vi "tailflickgui_v0.3.vi"() -> ()   [LabVIEW 2011]
uses:
  <vilib>/Utility/error.llb/DialogType.ctl
  <vilib>/Instr/_visa.llb/VISA Flush IO Buffer Mask.ctl
  <vilib>/Instr/_visa.llb/VISA Configure Serial Port (Instr).vi
  <vilib>/Utility/file.llb/Write To Spreadsheet File (string).vi
panel:
  in  "Start?":bool
  in  "End Experiments?":bool
  out "find list":string[](array[string])
  out "VISA resource name out":refnum<visa-resource-name>
  out "Lamp On":bool
  out "Elapsed Time (s)":dbl
  out "new file path (Not A Path if cancelled)":path
  in  "Sample Name":string="Mouse1"
  in  "Filename":path
  out "Start ms":u32
  out "Data Bits":u32
  in  "Arduino Port":refnum<visa-resource-name>
  in  "Baud Rate":dbl=19200.0
  out "USB Output":string
  out "error out":errorcluster
  in  "error in (no error)":errorcluster
  # "Important inputs and outputs for the user."
  # "Inputs and Outputs that should not need to be changed. They are for debugging."
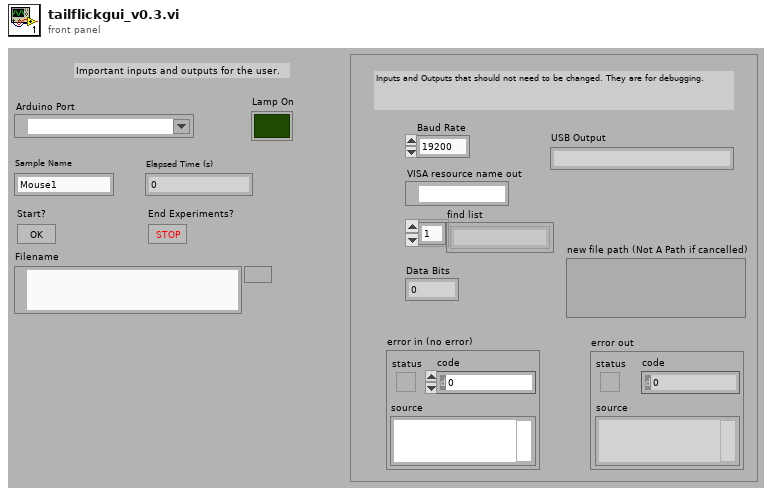
[diagram p1: front panel]
types:
  T1 = typedef "DialogType.ctl" = u16
  T2 = typedef "VISA Flush IO Buffer Mask.ctl" = u16
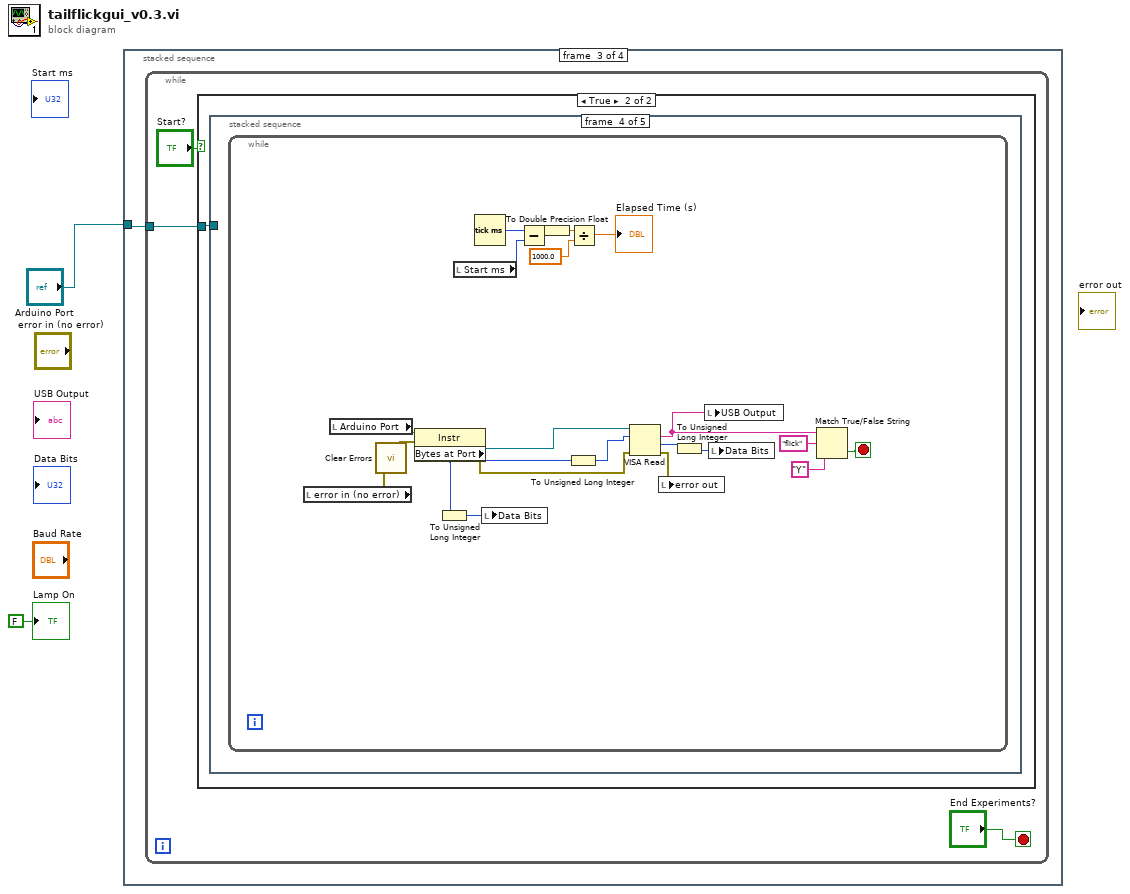
[diagram p0: block diagram]
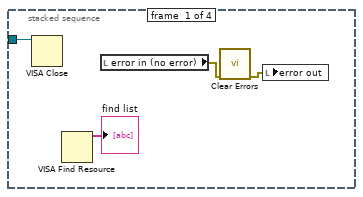
[diagram p2: hidden frame]
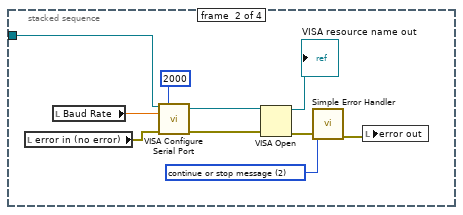
[diagram p3: hidden frame]
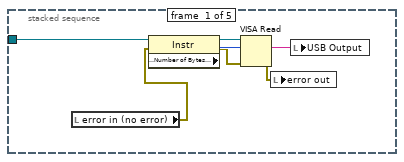
[diagram p5: hidden frame]
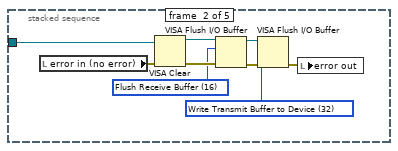
[diagram p6: hidden frame]
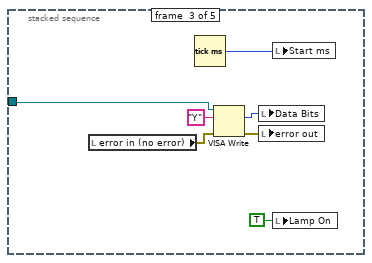
[diagram p7: hidden frame]
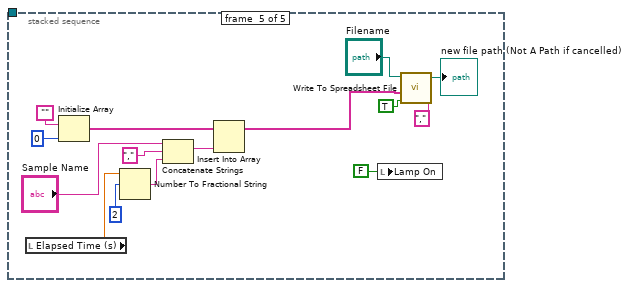
[diagram p8: hidden frame]
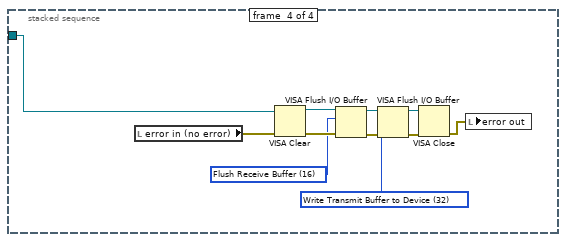
[diagram p9: hidden frame]
diagram:
  n1 = stacked-sequence {
    tunnel: "Arduino Port" -> [w4 w13 w17 w81]
    frame #0 {
      n2 = VISA Close(VISA resource name=w4) -> ()  [unwired: 1 in, 1 out]
      n3 = VISA Find Resource() -> (3:→"find list":string[])  [unwired: 3 in, 2 out]
      n4 = local read "error in (no error)"() -> (w6:errorcluster)
      n5 = call <vilib>:"Clear Errors.vi"("error in (no error)"=w6) -> ("error out"=w5:errorcluster)  [unwired: 6 in]
      n6 = local write "error out"(w5) -> ()
    }
    frame #1 {
      w8 = T1 2 items=["no dialog", "OK message", "continue or stop message", "OK message + warnings", "continue/stop + warnings"] ("type of dialog (OK msg:1)")
      n7 = local read "error in (no error)"() -> (w14:errorcluster)
      n8 = local read "Baud Rate"() -> (w16:dbl)
      n9 = call-poly "VISA Configure Serial Port"("VISA resource name"=w13, "timeout (10sec)"=u32 2000, "baud rate (9600)"=w16, "error in (no error)"=w14) -> ("VISA resource name out"=w12:refnum<visa-resource-name>, "error out"=w11:errorcluster)  [unwired: 10 in]
      n10 = VISA Open(error in (no error)=w11, VISA resource name=w12) -> (VISA resource name=→"VISA resource name out":refnum<visa-resource-name>, error out=w10:errorcluster)  [unwired: 3 in]
      n11 = call <vilib>:"Simple Error Handler.vi"("type of dialog (OK msg:1)"=w8, "error in (no error)"=w10) -> ("error out"=w9:errorcluster)  [unwired: 3 in, 4 out]
      n12 = local write "error out"(w9) -> ()
    }
    frame #2 {
      n13 = while {
        tunnel: w17 -> [w18]
        stop <- "End Experiments?" stop-if-true
        n14 = case shown="True" "Start?" {
          tunnel: w18 -> [_ w21]
          frame False {
          }
          frame True {
            n15 = stacked-sequence {
              tunnel: w21 -> [w25 w29 w40 _ _]
              frame #0 {
                n16 = local read "error in (no error)"() -> (w22:errorcluster)
                n17 = property class="Instr"(reference=w25, error in=w22) -> (reference out=w24:refnum<visa-resource-name>, error out=w23:errorcluster, "Serial Settings:Number of Bytes at Serial Port"=w26:u32)
                n18 = VISA Read(VISA resource name=w24, byte count=w26, error in (no error)=w23) -> (read buffer=w27:string, error out=w28:errorcluster)  [unwired: 2 out]
                n19 = local write "error out"(w28) -> ()
                n20 = local write "USB Output"(w27) -> ()
              }
              frame #1 {
                w33 = T2 32 items=["Flush Receive Buffer"=16, "Write Transmit Buffer to Device"=32, "Flush Receive Buffer (No I/O)"=64, "Flush Transmit Buffer"=128] ("Mask")
                w35 = T2 16 items=["Flush Receive Buffer"=16, "Write Transmit Buffer to Device"=32, "Flush Receive Buffer (No I/O)"=64, "Flush Transmit Buffer"=128] ("Mask")
                n21 = local read "error in (no error)"() -> (w30:errorcluster)
                n22 = VISA Clear(VISA resource name=w29, error in (no error)=w30) -> (VISA resource name out=w36:refnum<visa-resource-name>, error out=w37:errorcluster)
                n23 = VISA Flush I/O Buffer(VISA resource name=w36, mask (16)=w35, error in (no error)=w37) -> (VISA resource name out=w32:refnum<visa-resource-name>, error out=w34:errorcluster)
                n24 = VISA Flush I/O Buffer(VISA resource name=w32, mask (16)=w33, error in (no error)=w34) -> (error out=w31:errorcluster)  [unwired: 1 out]
                n25 = local write "error out"(w31) -> ()
              }
              frame #2 {
                n26 = local read "error in (no error)"() -> (w43:errorcluster)
                n27 = Tick Count (ms)() -> (millisecond timer value=w38:u32)
                n28 = VISA Write(VISA resource name=w40, write buffer="Y", error in (no error)=w43) -> (return count=w41:u32, error out=w42:errorcluster)  [unwired: 1 out]
                n29 = local write "Data Bits"(w41) -> ()
                n30 = local write "error out"(w42) -> ()
                n31 = local write "Start ms"(w38) -> ()
                n32 = local write "Lamp On"(TRUE) -> ()
              }
              frame #3 {
                n33 = while {
                  stop <- w60 stop-if-true
                  n34 = local read "error in (no error)"() -> (w56:errorcluster)
                  n35 = local read "Arduino Port"() -> (w55:refnum<visa-resource-name>)
                  n36 = call <vilib>:"Clear Errors.vi"("error in (no error)"=w56) -> ("error out"=w54:errorcluster)  [unwired: 6 in]
                  n37 = property class="Instr"(reference=w55, error in=w54) -> (reference out=w63:refnum<visa-resource-name>, error out=w61:errorcluster, "Bytes at Port"=w62:u32)
                  n38 = To Unsigned Long Integer(number=w62) -> (unsigned 32bit integer=w51:u32)
                  n39 = local read "Start ms"() -> (w48:u32)
                  n40 = Tick Count (ms)() -> (millisecond timer value=w50:u32)
                  n41 = local write "Data Bits"(w51) -> ()
                  n42 = Subtract(x=w50, y=w48) -> (x-y=w49:u32)
                  n43 = To Double Precision Float(number=w49) -> (double precision float=w45:dbl)
                  n44 = To Unsigned Long Integer(number=w62) -> (unsigned 32bit integer=w53:u32)
                  n45 = Divide(x=w45, y=1000.0) -> (x/y=→"Elapsed Time (s)":dbl)
                  n46 = VISA Read(VISA resource name=w63, byte count=w53, error in (no error)=w61) -> (read buffer=w64:string, return count=w59:u32, error out=w57:errorcluster)  [unwired: 1 out]
                  n47 = local write "error out"(w57) -> ()
                  n48 = To Unsigned Long Integer(number=w59) -> (unsigned 32bit integer=w52:u32)
                  n49 = local write "USB Output"(w64) -> ()
                  n50 = local write "Data Bits"(w52) -> ()
                  n51 = Match True/False String(2:"Y" ("false string"), 3:"flick" ("true string"), 4:w64) -> (0:w60:bool)  [unwired: 1 out]
                }
              }
              frame #4 {
                n52 = local read "Elapsed Time (s)"() -> (w68:dbl)
                n53 = Initialize Array("", 0 ("index")) -> (w74:string[])
                n54 = Number To Fractional String(number=w68, width (-)=i16 2 ("precision (6)")) -> (F-format string=w70:string)  [unwired: 2 in]
                n55 = Concatenate Strings("Sample Name", ",", w70) -> (w72:string)
                n56 = Insert Into Array(array=w74, new element=w72) -> (w67:string[])  [unwired: 1 in]
                n57 = local write "Lamp On"(FALSE ("Lamp On")) -> ()
                n58 = call-poly <vilib>:"Write To Spreadsheet File.vi"("delimiter (\\t)"="," ("delimiter (\\t)"), "append to file? (new file:F)"=TRUE, "1D data"=w67, "file path (dialog if empty)"="Filename") -> ("new file path (Not A Path if cancelled)"=→"new file path (Not A Path if cancelled)":path)  [unwired: 4 in]
              }
            }
          }
        }
      }
    }
    frame #3 {
      w87 = T2 32 items=["Flush Receive Buffer"=16, "Write Transmit Buffer to Device"=32, "Flush Receive Buffer (No I/O)"=64, "Flush Transmit Buffer"=128] ("Mask")
      w89 = T2 16 items=["Flush Receive Buffer"=16, "Write Transmit Buffer to Device"=32, "Flush Receive Buffer (No I/O)"=64, "Flush Transmit Buffer"=128] ("Mask")
      n59 = local read "error in (no error)"() -> (w85:errorcluster)
      n60 = VISA Clear(VISA resource name=w81, error in (no error)=w85) -> (VISA resource name out=w90:refnum<visa-resource-name>, error out=w91:errorcluster)
      n61 = VISA Flush I/O Buffer(VISA resource name=w90, mask (16)=w89, error in (no error)=w91) -> (VISA resource name out=w86:refnum<visa-resource-name>, error out=w88:errorcluster)
      n62 = VISA Flush I/O Buffer(VISA resource name=w86, mask (16)=w87, error in (no error)=w88) -> (VISA resource name out=w83:refnum<visa-resource-name>, error out=w84:errorcluster)
      n63 = VISA Close(VISA resource name=w83, error in (no error)=w84) -> (error out=w82:errorcluster)
      n64 = local write "error out"(w82) -> ()
    }
  }
  "Lamp On" <- FALSE ("Lamp On")
